vi "Track Used Subpanels.vi"(8 "error in (no error)":errorcluster, 10 "Used SubPanels":refnum<vi>[](array[refnum]), 11 "2DArrayManager in":refnum<class "2DArrayManager.lvclass">) -> (0 "error out":errorcluster, 3 "2DArrayManager out":refnum<class "2DArrayManager.lvclass">)   [LabVIEW 2020, in "OOPanel.lvlib" / "2DArrayManager.lvclass"]
uses:
  2DArrayManager.lvclass
  2DArrayManager.lvclass/2DArrayManager.ctl
  2DPanelBlank/2DPanelBlank.lvclass
  2DPanelBlank/State.ctl
  ArrayPanel/ArrayPanel.lvclass
  2DPanelBlank/2DPanelBlank.lvclass/2DPanelBlank.ctl
  Manager/Manager.lvclass
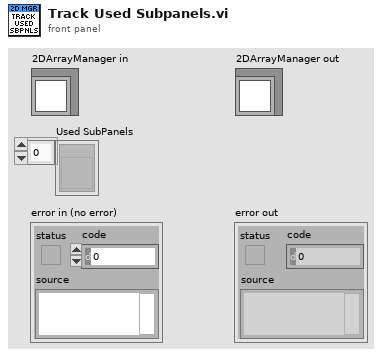
[diagram p1: front panel]
types:
  T1 = typedef "OOPanel.lvlib/2DPanelBlank.lvclass/State.ctl" = enum16{"New", "Idle", "Pool", "Used"}
  T2 = typedef "OOPanel.lvlib/2DPanelBlank.lvclass/Info.ctl" = cluster{"Index":T3, "State":T1, "Pull Count":i32}
  T3 = typedef "OOPanel.lvlib/2D Index.ctl" = cluster{"Row":i32, "Col":i32}
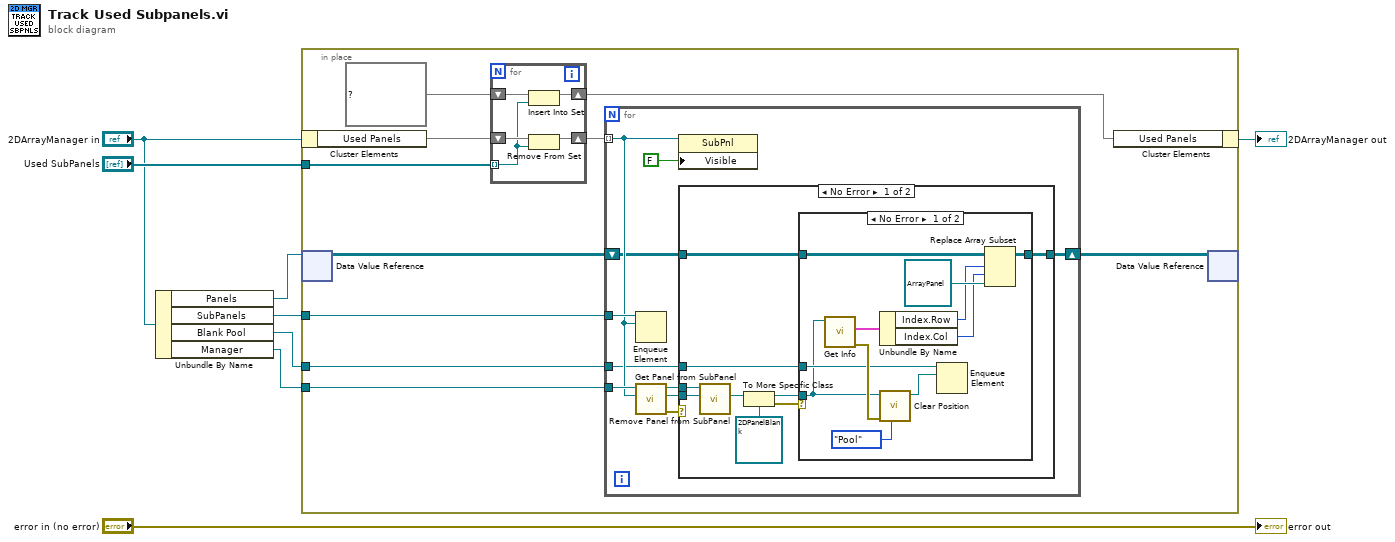
[diagram p0: block diagram]
diagram:
  n1 = Unbundle By Name("2DArrayManager in") -> ("Panels"=w1:refnum<data-value>, "SubPanels"=w4:refnum<queue>, "Blank Pool"=w2:refnum<queue>, "Manager"=w5:refnum<class "Manager.lvclass">)
  n2 = in-place {
    in-place-border: "Used SubPanels" -> [w17]
    in-place-border: w5 -> [w13]
    in-place-border: w4 -> [w12]
    in-place-border: w2 -> [w11]
    n3 = in-place-cluster #1("2DArrayManager in") -> ("Used Panels"=w18:set{refnum<vi>})
    n4 = in-place-dvr #2(w1) -> (w10:refnum<class "ArrayPanel.lvclass">[][])  [unwired: 1 out]
    n5 = for {
      tunnel: w17 -> [w52] mode=indexing
      shift-right: [w54] -> w14
      shift-left: w18 -> [w55]
      shift-right: [w51] -> w15
      shift-left: set{refnum<vi>} {} ("UI Refs.Used Panels") -> [w53]
      n6 = Insert Into Set(10:w52, 11:w53) -> (3:w51:set{refnum<vi>})  [unwired: 1 out]
      n7 = Remove From Set(10:w52, 11:w55) -> (3:w54:set{refnum<vi>})  [unwired: 1 out]
    }
    n8 = for {
      tunnel: w14 -> [w23] mode=indexing
      tunnel: w13 -> [w28]
      tunnel: w12 -> [w24]
      tunnel: w11 -> [w21]
      shift-right: [w19] -> w9
      shift-left: w10 -> [w20]
      n9 = Enqueue Element(queue=w24, element=w23) -> ()  [unwired: 2 in, 3 out]
      n10 = call "Get Panel from SubPanel.vi"("SubPanel"=w23, "Manager in"=w28) -> ("error out"=w25:errorcluster, "Panel"=w26:refnum<class "Panel.lvclass">, "Manager out"=w27:refnum<class "Manager.lvclass">)  [unwired: 6 in, 1 out]
      n11 = property class="SubPnl"(reference=w23, "Visible"=FALSE) -> ()  [unwired: 1 in, 2 out]
      n12 = case shown="No Error" w25 {
        tunnel: w27 -> [w33 _]
        tunnel: w26 -> [w32 _]
        tunnel: w21 -> [w34 _]
        tunnel: w20 -> [w30 w50]
        tunnel: [w29 w50] -> w19
        frame No Error {
          n13 = call "Remove Panel from SubPanel.vi"("Panel In"=w32, "Manager in"=w33) -> ("Panel"=w31:refnum<class "Panel.lvclass">)  [unwired: 7 in, 2 out]
          n14 = To More Specific Class(target class=refnum<class "2DPanelBlank.lvclass"> refnum ("OOPanel.lvlib:2DPanelBlank.lvclass"), reference=w31) -> (specific class reference=w35:refnum<class "2DPanelBlank.lvclass">, error out=w36:errorcluster)  [unwired: 1 in]
          n15 = case shown="No Error" w36 {
            tunnel: w35 -> [w43 _]
            tunnel: w34 -> [w47 _]
            tunnel: w30 -> [w46 w49]
            tunnel: [w45 w49] -> w29
            frame No Error {
              n16 = call "Get Info.vi"("2DPanelBlank in"=w43) -> ("error out"=w48:errorcluster, "Info"=w41:T2)  [unwired: 8 in, 1 out]
              n17 = Unbundle By Name(w41) -> ("Index.Row"=w40:i32, "Index.Col"=w39:i32)
              n18 = call "Clear Position.vi"("State"=State."Pool", "error in (no error)"=w48, "2DPanelBlank in"=w43) -> ("2DPanelBlank out"=w44:refnum<class "2DPanelBlank.lvclass">)  [unwired: 7 in, 1 out]
              n19 = Enqueue Element(queue=w47, element=w44) -> ()  [unwired: 2 in, 3 out]
              n20 = Replace Array Subset(array=w46, new element=refnum<class "ArrayPanel.lvclass"> refnum ("new element/subarray"), index (row)=w40, index (col)=w39) -> (w45:refnum<class "ArrayPanel.lvclass">[][])
            }
            frame Error {
            }
          }
        }
        frame Error {
        }
      }
    }
    n21 = in-place-cluster #1("Used Panels"=w15) -> (→"2DArrayManager out":refnum<class "2DArrayManager.lvclass">)
    n22 = in-place-dvr #2(w9) -> ()  [unwired: 2 out]
  }
  "error out" <- "error in (no error)"
